vi "SMU_Single Channel Meas_No Publish.vi"(7 "Meas_A_Level":dbl, 8 "error in (no error)":errorcluster, 10 "Pins":string[](array[string]), 11 "Semiconductor Module Context":T1) -> (0 "error Out":errorcluster, 2 "R Array":dbl[](array[numeric]), 3 "Semiconductor Module Context Out":T1)   [LabVIEW 2013]
uses:
  <vilib>/NI_TestStand_SemiconductorModule/NI_TestStand_Semiconductor_Module.lvlibp/PinMap/General/SemiconductorModuleContext.ctl
  <vilib>/NI_TestStand_SemiconductorModule/NI_TestStand_Semiconductor_Module.lvlibp/PinMap/DC Power/PinsToNIDCPowerSessions.vi
  <vilib>/NI_TestStand_SemiconductorModule/NI_TestStand_Semiconductor_Module.lvlibp
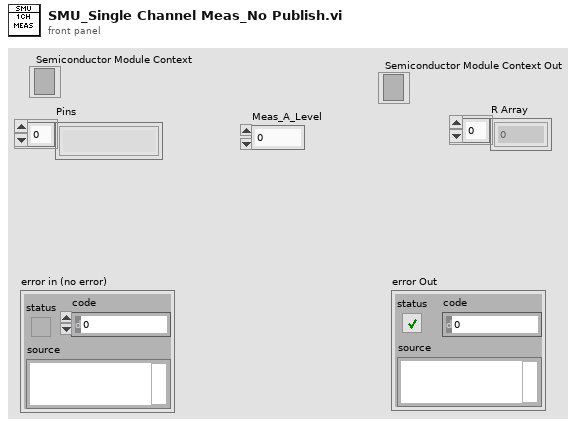
[diagram p1: front panel]
types:
  T1 = typedef "NI_TestStand_Semiconductor_Module.lvlibp/SemiconductorModuleContext.ctl" = refnum<k7>
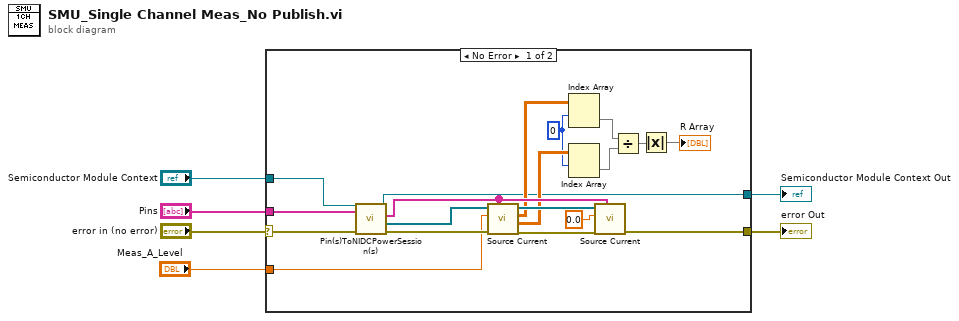
[diagram p0: block diagram]
diagram:
  n1 = case shown="No Error" "error in (no error)" {
    selector: "error in (no error)" -> [w25 w27]
    tunnel: "Semiconductor Module Context" -> [w23 w26]
    tunnel: "Pins" -> [w24 _]
    tunnel: [w10 w27] -> w3
    tunnel: [w9 w26] -> w2
    tunnel: "Meas_A_Level" -> [w11 _]
    frame No Error {
      w14 = 0 ("index (row)")
      n2 = call-poly <vilib>:"Pin(s)ToNIDCPowerSession(s).vi"("error in (no error)"=w25, "Pins"=w24, "Semiconductor Module Context"=w23) -> ("error out"=w20:errorcluster, "Instrument Sessions"=w21:refnum<k15>[], "Channel Lists"=w19:string[], "Semiconductor Module Context Out"=w9:T1)  [unwired: 4 in, 1 out]
      n3 = call "Source Current.vi"("Channel Lists"=w19, "error in (no error)"=w20, "current level"=w11, "Instrument Sessions In"=w21) -> ("error out"=w18:errorcluster, "current measurements"=w15:dbl[][], "voltage measurements"=w16:dbl[][], "Instrument Sessions Out"=w17:refnum<k15>[])  [unwired: 4 in]
      n4 = Index Array(array=w16, index (row)=w14) -> (element=w13:dbl[])  [unwired: 1 in]
      n5 = Index Array(array=w15, index (row)=w14) -> (element=w12:dbl[])  [unwired: 1 in]
      n6 = call "Source Current.vi"("Channel Lists"=w19, "error in (no error)"=w18, "current level"=0.0, "Instrument Sessions In"=w17) -> ("error out"=w10:errorcluster)  [unwired: 4 in, 3 out]
      n7 = Divide(x=w13, y=w12) -> (x/y=w8:dbl[])
      n8 = Absolute Value(x=w8) -> (abs(x)=→"R Array":dbl[])
    }
    frame Error {
    }
  }
  "error Out" <- w3
  "Semiconductor Module Context Out" <- w2
